vi "Set GUI Control.vi"(8 "error in (no error)":errorcluster, 10 "GUI Control":refnum<class "GUI Control.lvclass">, 11 "Console Reply Add Control in":refnum<class "Console Reply Add Control.lvclass">) -> (0 "error out":errorcluster, 3 "Console Reply Add Control out":refnum<class "Console Reply Add Control.lvclass">)   [LabVIEW 2015, in "Console Reply Add Control.lvclass"]
uses:
  Console Reply Add Control.lvclass
  GUI/GUI Controls/GUI Control/GUI Control.lvclass
  Console Reply Add Control.lvclass/Console Reply Add Control.ctl
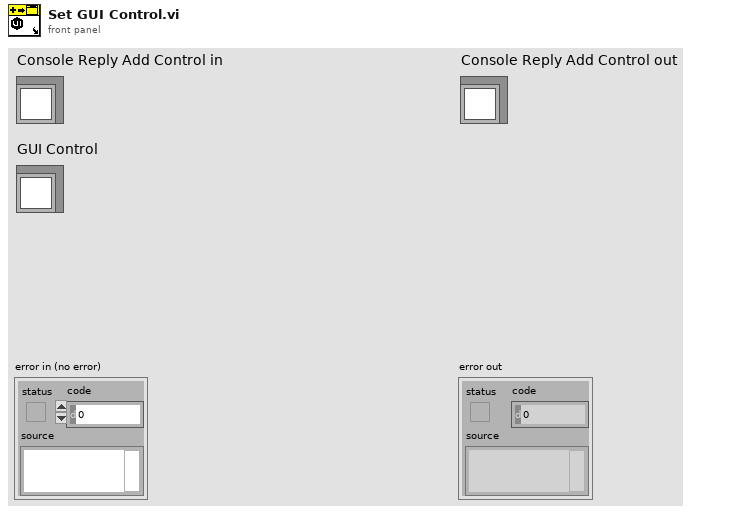
[diagram p1: front panel]
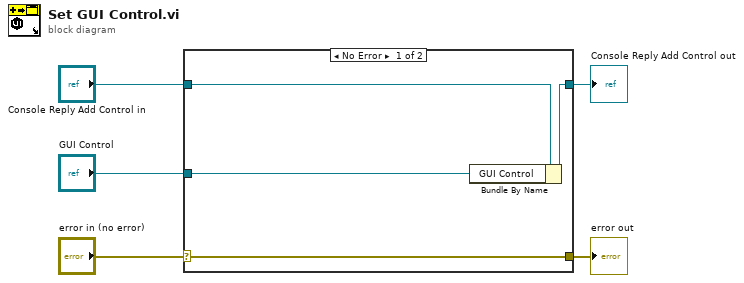
[diagram p0: block diagram]
diagram:
  n1 = case shown="No Error" "error in (no error)" {
    selector: "error in (no error)" -> [w9 w10]
    tunnel: [w9 w10] -> w4
    tunnel: [w7 w11] -> w2
    tunnel: "Console Reply Add Control in" -> [w8 w11]
    tunnel: "GUI Control" -> [w6 _]
    frame No Error {
      n2 = Bundle By Name(cluster=w8, "GUI Control"=w6) -> (w7:refnum<class "Console Reply Add Control.lvclass">)
    }
    frame Error {
    }
  }
  "error out" <- w4
  "Console Reply Add Control out" <- w2
